vi "array_find.vi"() -> ()   [LabVIEW 2024]
uses:
  Control 1.ctl
panel:
  in  "Search Element":dbl
  out "Index of Element":T1
  out "Array":dbl[](array[numeric])
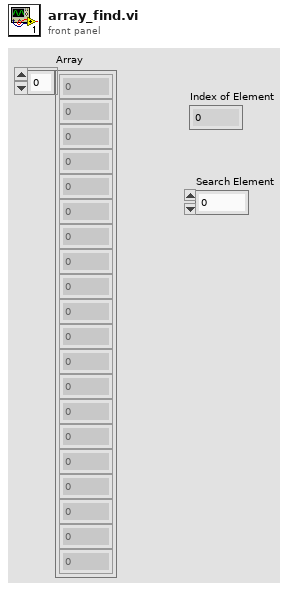
[diagram p1: front panel]
types:
  T1 = typedef "Control 1.ctl" = dbl
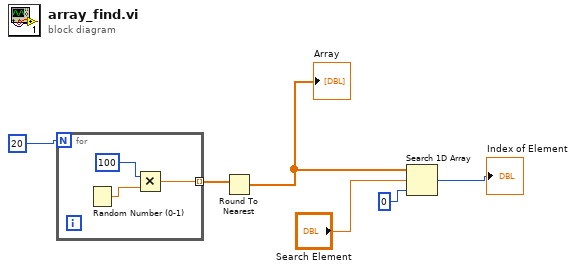
[diagram p0: block diagram]
diagram:
  n1 = for {
    N: 20 -> [_]
    tunnel: [w7] -> w5 mode=indexing
    n2 = Random Number (0-1)() -> (number: 0 to 1=w9:dbl)
    n3 = Multiply(x=100, y=w9) -> (x*y=w7:dbl)
  }
  n4 = Round To Nearest(number=w5) -> (nearest integer value=w4:dbl[])
  "Array" <- w4
  n5 = Search 1D Array(1D array=w4, element="Search Element", start index (0)=0) -> (index of element=→"Index of Element":i32)
